vi "SynapseAPI-Get Parameter Value.vi"(0 "URL":string="http://localhost:24414", 5 "Gizmo":string, 7 "Parameter":string, 11 "error in (no error)":errorcluster) -> (15 "error out":errorcluster)   [LabVIEW 2015]
uses:
  <vilib>/httpClient/LabVIEWHTTPClient.lvlib
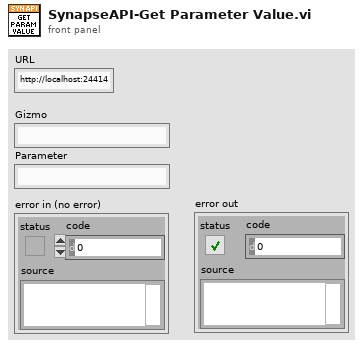
[diagram p1: front panel]
types:
  T1 = typedef "LabVIEWHTTPClient.lvlib/ClientHandle.ctl" = refnum<k1>
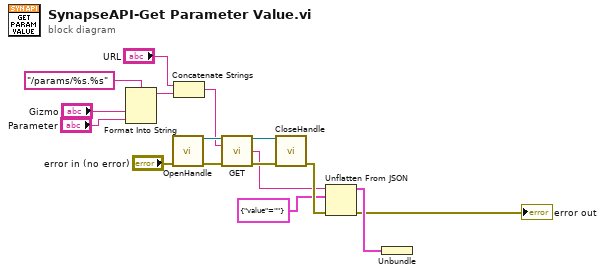
[diagram p0: block diagram]
diagram:
  n1 = Format Into String(format string="/params/%s.%s", "Gizmo", "Parameter") -> (resulting string=w5:string)  [unwired: 2 in, 1 out]
  n2 = call <vilib>:"OpenHandle.vi"("error in (no error)"="error in (no error)") -> ("client handle out"=w14:T1, "error out"=w13:errorcluster)  [unwired: 13 in]
  n3 = Concatenate Strings("URL", w5) -> (w7:string)
  n4 = call <vilib>:"GET.vi"("client handle"=w14, "url"=w7, "error in (no error)"=w13) -> ("client handle out"=w15:T1, "body"=w10:string, "error out"=w16:errorcluster)  [unwired: 9 in, 1 out]
  n5 = call <vilib>:"CloseHandle.vi"("client handle"=w15, "error in (no error)"=w16) -> ("error out"=w12:errorcluster)  [unwired: 13 in]
  n6 = Unflatten From JSON(JSON string=w10, type and defaults=cluster{"value":string} {"value"=""} ("Cluster"), error in (no error)=w12) -> (value=w8:cluster{"value":string}, error out=→"error out":errorcluster)  [unwired: 4 in]
  n7 = Unbundle(w8) -> ()  [unwired: 1 out]
